vi "Bind Insert Update Command Values.vi"(8 "Error In (no error)":errorcluster, 10 "Record":variant, 11 "SQL Statement In":refnum<class "SQL Statement.lvclass">) -> (0 "Error Out":errorcluster, 3 "SQL Statement Out":refnum<class "SQL Statement.lvclass">)   [LabVIEW 2023, in "SQLite DB Operator.lvclass"]
uses:
  SQLite DB Operator.lvclass
  <vilib>/drjdpowell/SQLite Library/SQL Statement/SQL Statement.lvclass
  DB Records/Expenses Tracker Record/Public/Ctrls/Category.ctl
  <vilib>/drjdpowell/SQLite Library/SQL Statement/SQL Statement.lvclass/SQL Statement.ctl
  DB Records/Expenses Tracker Record/Public/Ctrls/Transaction.ctl
  <vilib>/drjdpowell/SQLite Library/SQL Statement/Bind Text.vi
  <vilib>/drjdpowell/SQLite Library/SQL Statement/Bind Null.vi
  <vilib>/drjdpowell/SQLite Library/SQL Statement/Bind Integer.vi
  <vilib>/drjdpowell/SQLite Library/SQL Statement/Bind Real.vi
  <vilib>/drjdpowell/SQLite Library/SQL Statement/Bind Timestamp (Real).vi
  <vilib>/drjdpowell/SQLite Library/SQL Statement/Error Message.vi
  SQLite DB Operator.lvclass/SQLite DB Operator.ctl
  DB Records/Expenses Tracker Record/Expenses Tracker Record.lvclass
  <vilib>/Utility/Data Type/NI_Data Type.lvlib
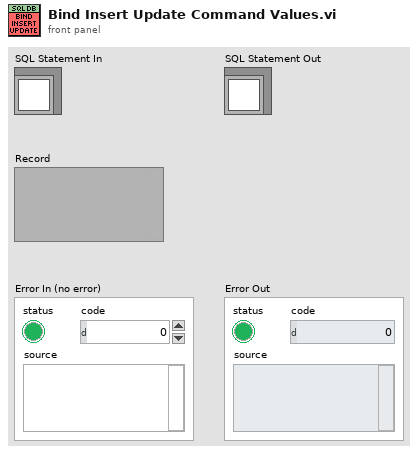
[diagram p1: front panel]
types:
  T1 = typedef "Expenses Tracker Record.lvclass/Category.ctl" = cluster{"ID":u32, "Name":string}
  T2 = typedef "Expenses Tracker Record.lvclass/Transaction.ctl" = cluster{"ID":u32, "Name":string, "Is_income":bool, "Value":dbl, "Amount":dbl, "Total":dbl, "Date_of_entry":timestamp, "Date":timestamp, "Last_update":timestamp, "Category":u32, "Subcategory":u32, "Cycle":u32, "Description":string}
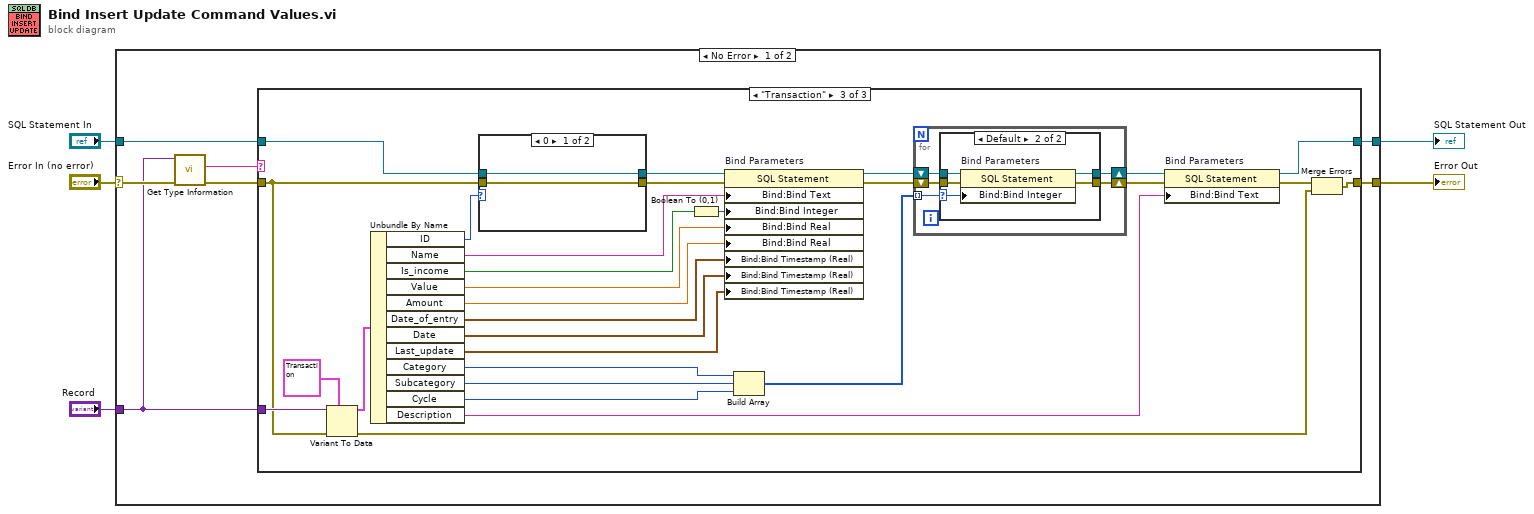
[diagram p0: block diagram]
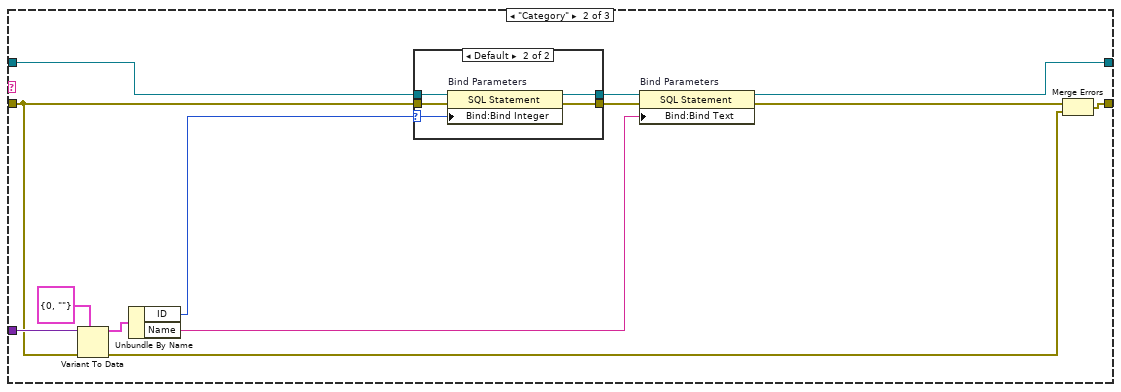
[diagram p3: hidden frame]
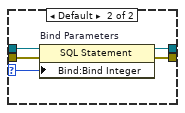
[diagram p5: hidden frame]
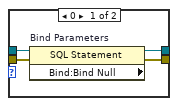
[diagram p6: hidden frame]
diagram:
  n1 = case shown="No Error" "Error In (no error)" {
    selector: "Error In (no error)" -> [w9 w85]
    tunnel: "SQL Statement In" -> [w12 w86]
    tunnel: [w11 w85] -> w4
    tunnel: [w10 w86] -> w3
    tunnel: "Record" -> [w8 _]
    frame No Error {
      n2 = call <vilib>:"Get Type Information.vi"("error in (no error)"=w9, "variant"=w8) -> ("error out"=w6:errorcluster, "name"=w7:string)  [unwired: 5 in, 3 out]
      n3 = case shown="\"Transaction\"" w7 {
        tunnel: w8 -> [_ w27 w63]
        tunnel: [w13 w26 w45] -> w10
        tunnel: [w14 w21 w59] -> w11
        tunnel: w12 -> [w13 w16 w38]
        tunnel: w6 -> [w14 w19 w39]
        frame Default {
        }
        frame "Category" {
          n4 = Variant To Data(error in=w19, type=T1 {"ID"=0, "Name"=""} ("Category"), Variant=w27) -> (data=w24:T1, error out=w20:errorcluster)
          n5 = Unbundle By Name(w24) -> ("ID"=w15:u32, "Name"=w22:string)
          n6 = case shown="Default" w15 {
            selector: w15 -> [_ w30]
            tunnel: w19 -> [w28 w34]
            tunnel: [w28 w33] -> w18
            tunnel: [w29 w32] -> w17
            tunnel: w16 -> [w29 w31]
            frame 0 {
            }
            frame Default {
              n7 = property on="Bind Parameters" class="SQL Statement"(reference=w31, error in=w34, "Bind:Bind Integer"=w30) -> (reference out=w32:refnum<class "SQL Statement.lvclass">, error out=w33:errorcluster)
            }
          }
          n8 = property on="Bind Parameters" class="SQL Statement"(reference=w17, error in=w18, "Bind:Bind Text"=w22) -> (reference out=w26:refnum<class "SQL Statement.lvclass">, error out=w25:errorcluster)
          n9 = Merge Errors(w25, w20) -> (w21:errorcluster)
        }
        frame "Transaction" {
          n10 = Variant To Data(error in=w39, type=T2 {"ID"=0, "Name"="", "Is_income"=FALSE, "Value"=0.0, "Amount"=0.0, "Total"=0.0, "Date_of_entry"=timestamp(0 s since 1904-01-01), "Date"=timestamp(0 s since 1904-01-01), "Last_update"=timestamp(0 s since 1904-01-01), "Category"=0, "Subcategory"=0, "Cycle"=0, "Description"=""} ("Transaction"), Variant=w63) -> (data=w62:T2, error out=w58:errorcluster)
          n11 = Unbundle By Name(w62) -> ("ID"=w35:u32, "Name"=w60:string, "Is_income"=w52:bool, "Value"=w56:dbl, "Amount"=w57:dbl, "Date_of_entry"=w55:timestamp, "Date"=w54:timestamp, "Last_update"=w53:timestamp, "Category"=w43:u32, "Subcategory"=w42:u32, "Cycle"=w41:u32, "Description"=w44:string)
          n12 = case shown="0" w35 {
            selector: w35 -> [_ w66]
            tunnel: w39 -> [w64 w70]
            tunnel: w38 -> [w65 w69]
            tunnel: [w64 w68] -> w37
            tunnel: [w65 w67] -> w36
            frame 0 {
            }
            frame Default {
              n13 = property on="Bind Parameters" class="SQL Statement"(reference=w69, error in=w70, "Bind:Bind Integer"=w66) -> (reference out=w67:refnum<class "SQL Statement.lvclass">, error out=w68:errorcluster)
            }
          }
          n14 = Boolean To (0,1)(Boolean=w52) -> (0, 1=w51:i16)
          n15 = property on="Bind Parameters" class="SQL Statement"(reference=w36, error in=w37, "Bind:Bind Text"=w60, "Bind:Bind Integer"=w51, "Bind:Bind Real"=w56, "Bind:Bind Real"=w57, "Bind:Bind Timestamp (Real)"=w55, "Bind:Bind Timestamp (Real)"=w54, "Bind:Bind Timestamp (Real)"=w53) -> (reference out=w49:refnum<class "SQL Statement.lvclass">, error out=w50:errorcluster)
          n16 = Build Array(w43, w42, w41) -> (w40:u32[])
          n17 = for {
            shift-right: [w72] -> w47
            shift-left: w50 -> [w75]
            shift-right: [w73] -> w48
            shift-left: w49 -> [w74]
            tunnel: w40 -> [w71] mode=indexing
            n18 = case shown="Default" w71 {
              selector: w71 -> [_ w80]
              tunnel: w75 -> [w79 w84]
              tunnel: w74 -> [w78 w83]
              tunnel: [w77 w82] -> w73
              tunnel: [w76 w81] -> w72
              frame 0 {
                n19 = property on="Bind Parameters" class="SQL Statement" props=["Bind:Bind Null"](reference=w78, error in=w79) -> (reference out=w77:refnum<class "SQL Statement.lvclass">, error out=w76:errorcluster)  [unwired: 1 out]
              }
              frame Default {
                n20 = property on="Bind Parameters" class="SQL Statement"(reference=w83, error in=w84, "Bind:Bind Integer"=w80) -> (reference out=w82:refnum<class "SQL Statement.lvclass">, error out=w81:errorcluster)
              }
            }
          }
          n21 = property on="Bind Parameters" class="SQL Statement"(reference=w48, error in=w47, "Bind:Bind Text"=w44) -> (reference out=w45:refnum<class "SQL Statement.lvclass">, error out=w46:errorcluster)
          n22 = Merge Errors(w46, w58) -> (w59:errorcluster)
        }
      }
    }
    frame Error {
    }
  }
  "Error Out" <- w4
  "SQL Statement Out" <- w3
